vi "Read state.vi"(8 "error in (no error)":errorcluster, 11 "Master CR in":refnum<class "Master CR.lvclass">) -> (0 "error out":errorcluster, 2 "state":T1=enum."configure", 3 "Master CR out":refnum<class "Master CR.lvclass">)   [LabVIEW 2021, in "Master CR.lvclass"]
uses:
  Master CR.lvclass
  ctl/CR_Core_State.ctl
  Master CR.lvclass/Master CR.ctl
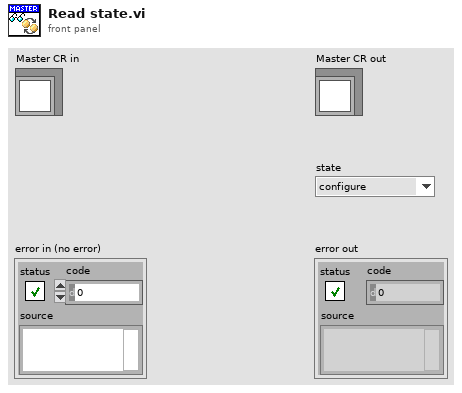
[diagram p1: front panel]
types:
  T1 = typedef "Master CR.lvclass/CR_Core_State.ctl" = enum8{"initialization", "redefine", "standby", "ping", "connect", "wait to reconnect", "wait to reset timeout", "configure", "requests", "close connection", "stop"}
  T2 = typedef "Master CR.lvclass/Master CR state.ctl" = cluster{"state":T1, "enable":bool, "write enable":bool, "connect":bool, "errors":i32, "Run":bool, "Write":bool, "Stop":bool}
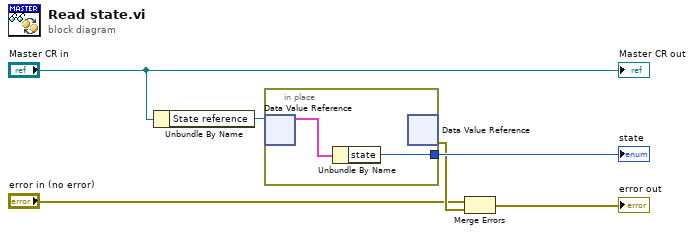
[diagram p0: block diagram]
diagram:
  n1 = Unbundle By Name("Master CR in") -> ("State reference"=w3:refnum<data-value>)
  n2 = in-place {
    in-place-border: [w8] -> w4
    n3 = in-place-dvr #1(w3) -> (w7:T2)  [unwired: 1 out]
    n4 = Unbundle By Name(w7) -> ("state"=w8:T1)
    n5 = in-place-dvr #1() -> (w2:errorcluster)  [unwired: 1 in, 1 out]
  }
  "state" <- w4
  n6 = Merge Errors("error in (no error)", w2) -> (→"error out":errorcluster)
  "Master CR out" <- "Master CR in"
